vi "Initialize Log.vi"(8 "error in (no error)":errorcluster, 11 "Json Logger in":refnum<class "Json Logger.lvclass">) -> (0 "error out":errorcluster, 3 "Json Logger out":refnum<class "Json Logger.lvclass">)   [LabVIEW 2021, in "Json Logger.lvclass"]
uses:
  Json Logger.lvclass
  <vilib>/gRPC/Generated APIs/ni/measurementlink/discovery/v1/RPC Messages/ni_measurementlink_discovery_v1_ResolveServiceRequest.ctl
  Json Logger.lvclass/Json Logger.ctl
  <vilib>/gRPC/Generated APIs/ni/measurementlink/discovery/v1/ni.measurementlink.discovery.v1.api.lvlib
  <vilib>/Plug-In SDKs/Clients/Discovery V1/NI Discovery V1 Client.lvlib
  log_measurement_client/log_measurement_client.lvlib
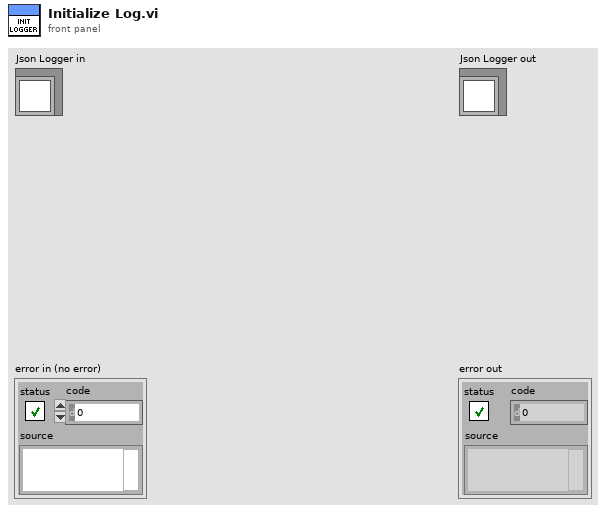
[diagram p1: front panel]
types:
  T1 = typedef "ni.measurementlink.discovery.v1.api.lvlib/ni_measurementlink_discovery_v1_ResolveServiceRequest.ctl" = cluster{"provided_interface":string, "service_class":string, "deployment_target":string, "version":string}
  T2 = typedef "ni.measurementlink.discovery.v1.api.lvlib/ni_measurementlink_discovery_v1_ServiceLocation.ctl" = cluster{"location":string, "insecure_port":string, "ssl_authenticated_port":string}
  T3 = typedef "grpc-lvsupport-release.lvlib/grpcId.ctl" = u64
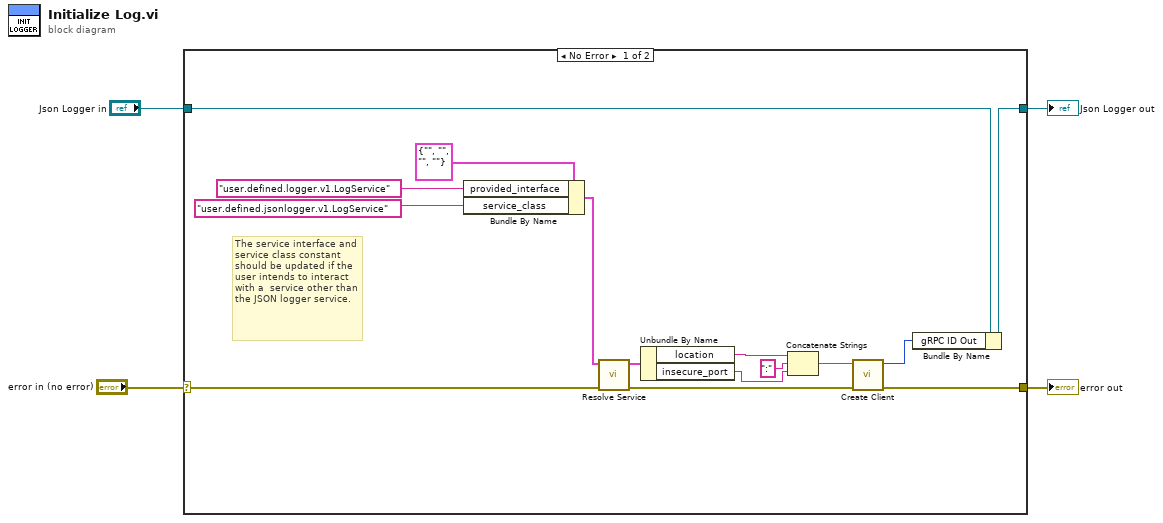
[diagram p0: block diagram]
diagram:
  n1 = case shown="No Error" "error in (no error)" {
    selector: "error in (no error)" -> [w8 w21]
    tunnel: [w7 w21] -> w3
    tunnel: [w6 w20] -> w1
    tunnel: "Json Logger in" -> [w19 w20]
    frame No Error {
      # "The service interface and service class constant should be updated if the user intends to interact with a  service other than the JSON logger service."
      n2 = Bundle By Name(cluster=T1 {"provided_interface"="", "service_class"="", "deployment_target"="", "version"=""} ("request data"), "provided_interface"="user.defined.logger.v1.LogService", "service_class"="user.defined.jsonlogger.v1.LogService") -> (w9:T1)
      n3 = call <vilib>:"Resolve Service.vi"("error in"=w8, "request data"=w9) -> ("error out"=w11:errorcluster, "response data"=w15:T2)  [unwired: 8 in]
      n4 = Unbundle By Name(w15) -> ("location"=w14:string, "insecure_port"=w12:string)
      n5 = Concatenate Strings(w14, ":" ("string"), w12) -> (w10:string)
      n6 = call "Create Client.vi"("error in"=w11, "address"=w10) -> ("error out"=w7:errorcluster, "gRPC ID Out"=w5:T3)  [unwired: 8 in]
      n7 = Bundle By Name(cluster=w19, "gRPC ID Out"=w5) -> (w6:refnum<class "Json Logger.lvclass">)
    }
    frame Error {
    }
  }
  "error out" <- w3
  "Json Logger out" <- w1
